vi "Workshop Exercise 3 Solution.vi"() -> ()   [LabVIEW 2019]
uses:
  <vilib>/ptbypt/NI_PtbyPt.lvlib
panel:
  out "Queue Loop Rate (ms)":dbl(knob) scale=0.0..100.0
  out "Local Variable Loop Rate (ms)":dbl(knob) scale=0.0..100.0
  out "Producer Loop Rate (ms)":dbl(knob) scale=0.0..100.0
  in  "Local Variable Loop Speed":u16(ring)=25 items=["Producer Loop Speed"=25, "Max. Speed"=0, "Twice as Producer"=12, "Half as Producer"=50, "1/10 as Producer"=250]
  in  "Queue Loop Speed":u16(ring)=25 items=["Producer Loop Speed"=25, "Max. Speed"=0, "Twice Producer Speed"=12, "Half Producer Speed"=50, "1/10 as Producer"=250]
  in  "Stop":bool
  out "Local Variable Loop":dbl(graph) caption="Local Variables Consumer Chart"
  out "Queue Loop":dbl(graph)=-9.510565162951542 caption="Queues Consumer Chart"
  out "Producer Loop":dbl(graph) caption="Producer Loop Chart"
  # "Producer Loop"
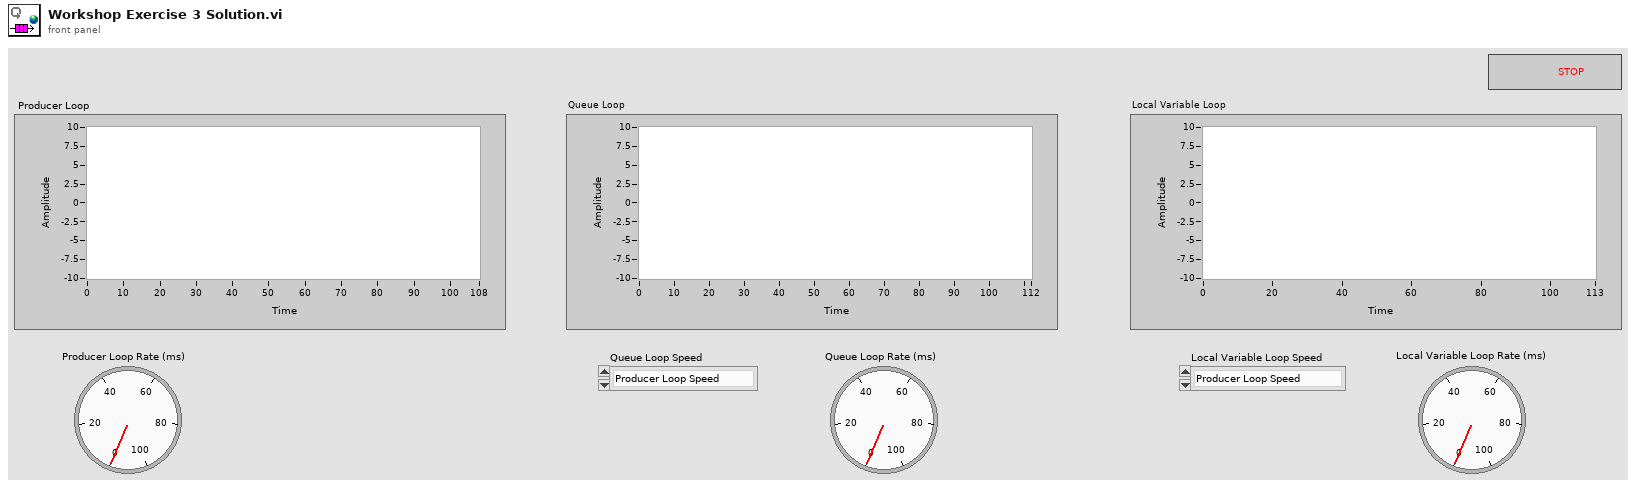
[diagram p1: front panel]
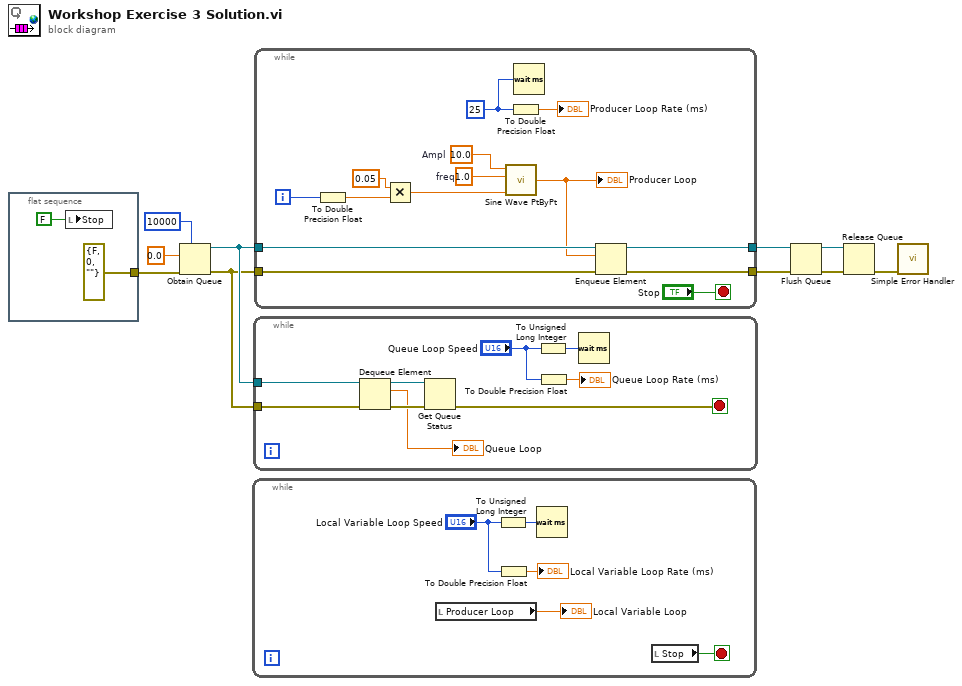
[diagram p0: block diagram]
diagram:
  n1 = flat-sequence {
    tunnel: [errorcluster {"status"=FALSE, "code"=0, "source"=""} ("error constant")] -> w5
    frame #0 {
      n2 = local write "Stop"(FALSE ("stop")) -> ()
    }
  }
  n3 = Obtain Queue(max queue size (-1, unlimited)=10000 ("max queue size"), element data type=0.0 ("Data Type"), error in (no error)=w5) -> (queue out=w9:refnum<queue>, error out=w8:errorcluster)  [unwired: 2 in, 1 out]
  n4 = while {
    stop <- w17 stop-if-true
    # "Local Variable Consumer Loop"
    n5 = local read "Producer Loop"() -> (→"Local Variable Loop":dbl)
    n6 = To Unsigned Long Integer(number="Local Variable Loop Speed") -> (unsigned 32bit integer=w15:u32)
    n7 = To Double Precision Float(number="Local Variable Loop Speed") -> (double precision float=→"Local Variable Loop Rate (ms)":dbl)
    n8 = Wait (ms)(milliseconds to wait=w15) -> ()  [unwired: 1 out]
    n9 = local read "Stop"() -> (w17:bool)
  }
  n10 = while {
    tunnel: w9 -> [w24]
    tunnel: w8 -> [w23]
    stop <- w22 stop-if-true
    # "Queue Consumer Loop"
    n11 = Dequeue Element(queue=w24, error in (no error)=w23) -> (queue out=w26:refnum<queue>, element=→"Queue Loop":dbl, error out=w25:errorcluster)  [unwired: 2 out]
    n12 = Get Queue Status(queue=w26, error in (no error)=w25) -> (error out=w22:errorcluster)  [unwired: 1 in, 7 out]
    n13 = To Unsigned Long Integer(number="Queue Loop Speed") -> (unsigned 32bit integer=w20:u32)
    n14 = To Double Precision Float(number="Queue Loop Speed") -> (double precision float=→"Queue Loop Rate (ms)":dbl)
    n15 = Wait (ms)(milliseconds to wait=w20) -> ()  [unwired: 1 out]
  }
  n16 = while {
    tunnel: w9 -> [w37]
    tunnel: w8 -> [w36]
    tunnel: [w39] -> w2
    tunnel: [w38] -> w7
    i -> [w34]
    stop <- "Stop" stop-if-true
    w30 = 1.0  # freq
    w31 = 10.0  # Ampl
    w33 = u32 25 ("milliseconds to wait")
    # "Producer Loop"
    n17 = To Double Precision Float(number=w34) -> (double precision float=w27:dbl)
    n18 = Multiply(x=0.05 ("milliseconds to wait"), y=w27) -> (x*y=w28:dbl)
    n19 = call <vilib>:"Sine Wave PtByPt.vi"("time"=w28, "frequency"=w30, "amplitude"=w31) -> ("sine wave"=w35:dbl)  [unwired: 1 in]
    "Producer Loop" <- w35
    n20 = To Double Precision Float(number=w33) -> (double precision float=→"Producer Loop Rate (ms)":dbl)
    n21 = Wait (ms)(milliseconds to wait=w33) -> ()  [unwired: 1 out]
    n22 = Enqueue Element(queue=w37, element=w35, error in (no error)=w36) -> (queue out=w38:refnum<queue>, error out=w39:errorcluster)  [unwired: 2 out]
  }
  n23 = Flush Queue(queue=w7, error in (no error)=w2) -> (queue out=w3:refnum<queue>, error out=w1:errorcluster)  [unwired: 1 out]
  n24 = Release Queue(queue=w3, error in (no error)=w1) -> (error out=w4:errorcluster)  [unwired: 1 in, 2 out]
  n25 = call <vilib>:"Simple Error Handler.vi"("error in (no error)"=w4) -> ()  [unwired: 2 in, 7 out]
